vi "Setup_Environment.vi"() -> (0 "First Time":bool)   [LabVIEW 2010]
uses:
  File/Setup_Filetype.ctl
  Globals/Meas_global.vi
panel:
  out "error string":string
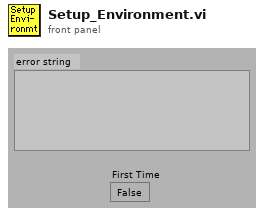
[diagram p1: front panel]
types:
  T1 = typedef "Setup_Filetype.ctl" = enum16{"Measurement Setups", "Calibration Setups", "General", "Results File Plotter Setups", "Speed Calib Tweaks"}
  T2 = cluster{"Start Index":i32, "End Index":i32, "Smoothing":enum16{"Linear", "Logarithmic"}, "Number of smoothed estimates":i32, "X axis":cluster{"Mapping":u16, "Format":u16}, "Y axis":cluster{"Mapping":u16, "Format":u16}, "Use Whole Input Array?":bool}[]
  T3 = cluster{"Start Index":i32, "End Index":i32, "Smoothing":enum16{"Linear", "Logarithmic"}, "Number of smoothed estimates":i32, "X axis":cluster{"Mapping":u16, "Format":u16}, "Y axis":cluster{"Mapping":u16, "Format":u16}, "Use Whole Input Array?":bool}
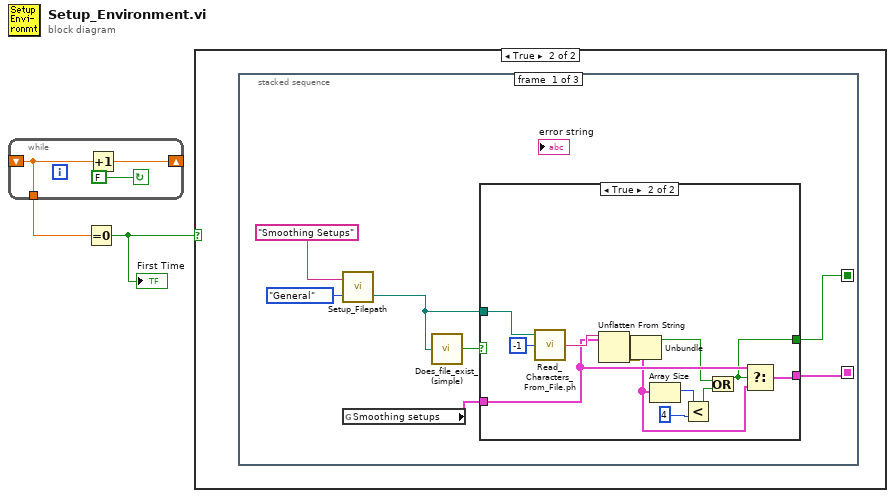
[diagram p0: block diagram]
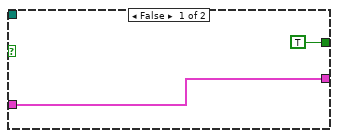
[diagram p3: hidden frame]
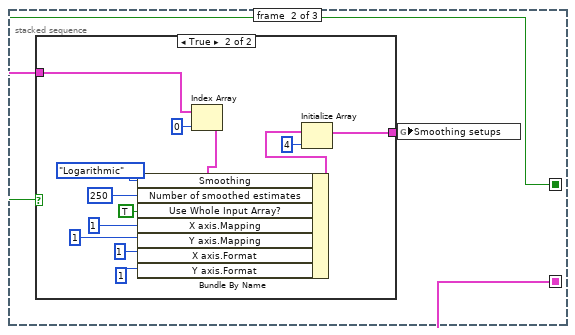
[diagram p4: hidden frame]
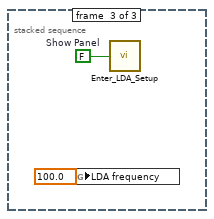
[diagram p6: hidden frame]
diagram:
  n1 = while {
    tunnel: [w5] -> w2
    shift-left: _ -> [w5]
    shift-right: [w4] -> _
    stop <- FALSE continue-if-true
    n2 = Increment(x=w5) -> (x+1=w4:dbl)
  }
  n3 = Equal To 0?(x=w2) -> (x = 0?=w1:bool)
  "First Time" <- w1
  n4 = case shown="True" w1 {
    frame False {
    }
    frame True {
      n5 = stacked-sequence {
        seq-local: [w10 _ _] -> [_ w29 _]
        seq-local: [w9 _ _] -> [_ w28 _]
        frame #0 {
          n6 = call "Setup_Filepath.vi"("Setup File Type"=Setup_Filetype."General", "Filename in"="Smoothing Setups" ("Substring")) -> ("Filename Out"=w6:path)  [unwired: 1 out]
          n7 = global read "Meas_global.vi" "Smoothing setups"() -> (w11:T2)
          n8 = call "Does_file_exist_(simple).vi"("Pathname"=w6) -> ("exists?"=w12:bool)
          n9 = case shown="True" w12 {
            tunnel: w6 -> [_ w25]
            tunnel: w11 -> [w14 w23]
            tunnel: [TRUE ("err") w16] -> w10
            tunnel: [w14 w22] -> w9
            frame False {
            }
            frame True {
              n10 = call "Read_Characters_From_File.ph.vi"("file path (dialog if empty)"=w25, "number of characters (all:-1)"=-1) -> ("character string"=w26:string)  [unwired: 7 out]
              n11 = Unflatten From String(type=w23, binary string=w26) -> (value=w17:T2, error out=w15:errorcluster)  [unwired: 1 in, 3 out]
              n12 = Unbundle(w15) -> ("status"=w18:bool)  [unwired: 2 out]
              n13 = Array Size(array=w17) -> (size(s)=w21:i32)
              n14 = Less?(x=w21, y=4) -> (x < y?=w19:bool)
              n15 = Or(x=w18, y=w19) -> (x .or. y?=w16:bool)
              n16 = Select(t=w23, s=w16, f=w17) -> (s? t:f=w22:T2)
            }
          }
        }
        frame #1 {
          n17 = case shown="True" w29 {
            tunnel: [w30 w40] -> w27
            tunnel: w28 -> [w30 w33]
            frame False {
            }
            frame True {
              n18 = Index Array(array=w33, index=0 ("Index")) -> (element=w41:T3)
              n19 = Bundle By Name(cluster=w41, "Smoothing"=enum16{"Linear", "Logarithmic"}."Logarithmic" ("Bundle Element"), "Number of smoothed estimates"=250 ("Bundle Element"), "Use Whole Input Array?"=TRUE ("Bundle Element"), "X axis.Mapping"=u16 1 ("Bundle Element"), "Y axis.Mapping"=u16 1 ("Bundle Element"), "X axis.Format"=u16 1 ("Bundle Element"), "Y axis.Format"=u16 1 ("Bundle Element")) -> (w34:T3)
              n20 = Initialize Array(w34, 4) -> (w40:T2)
            }
          }
          n21 = global write "Meas_global.vi" "Smoothing setups"(w27) -> ()
        }
        frame #2 {
          w44 = FALSE  # Show Panel
          n22 = global write "Meas_global.vi" "LDA frequency"(100.0 ("LDA frequency")) -> ()
          n23 = call "Enter_LDA_Setup.vi"("Show Panel"=w44) -> ()
        }
      }
    }
  }
